vi "chaos crest cu cmd.vi"(7 "args":string, 9 "cmd":string, 10 "cuname":string, 11 "handleConnection":u32) -> (3 "nok":i32)   [LabVIEW 2014, in "libcommon-crest.lvlib"]
doc: "int chaos_crest_cu_cmd(chaos_crest_handle_t h,const char*cuname,const char*cmd,const char* args);"
uses:
  libcommon-crest.lvlib
  chaos-i686-dynamic-release/lib/libcommon-crest.so
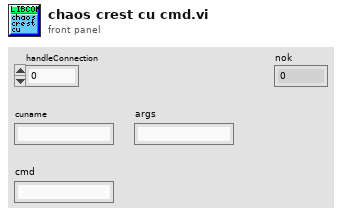
[diagram p1: front panel]
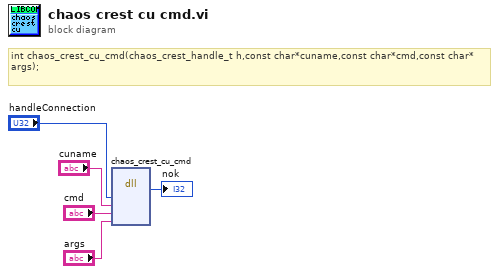
[diagram p0: block diagram]
diagram:
  # "int chaos_crest_cu_cmd(chaos_crest_handle_t h,const char*cuname,const char*cmd,const char* args);"
  n1 = dll-call lib="home/chaos/chaos_bundle/chaos-i686-dynamic-release/lib/libcommon-crest.*" fn="chaos_crest_cu_cmd"("handleConnection"="handleConnection", "cuname"="cuname", "cmd"="cmd", "args"="args") -> (→"nok":i32)  [unwired: 7 in, 2 out]
